vi "ctiSoubor.vi"(8 "PrecistSoubor":bool, 11 "Který soubor chcete otevřít?":path) -> (0 "vystupniError":errorcluster, 2 "Časové razítko souboru:":string, 3 "data":waveform(dbl)[](array[waveform]))   [LabVIEW 2018]
panel:
  # "Vstupy:"
  # "Výstupy:"
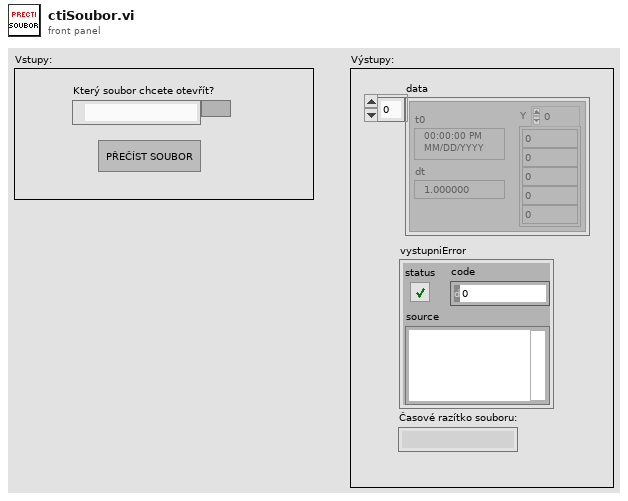
[diagram p1: front panel]
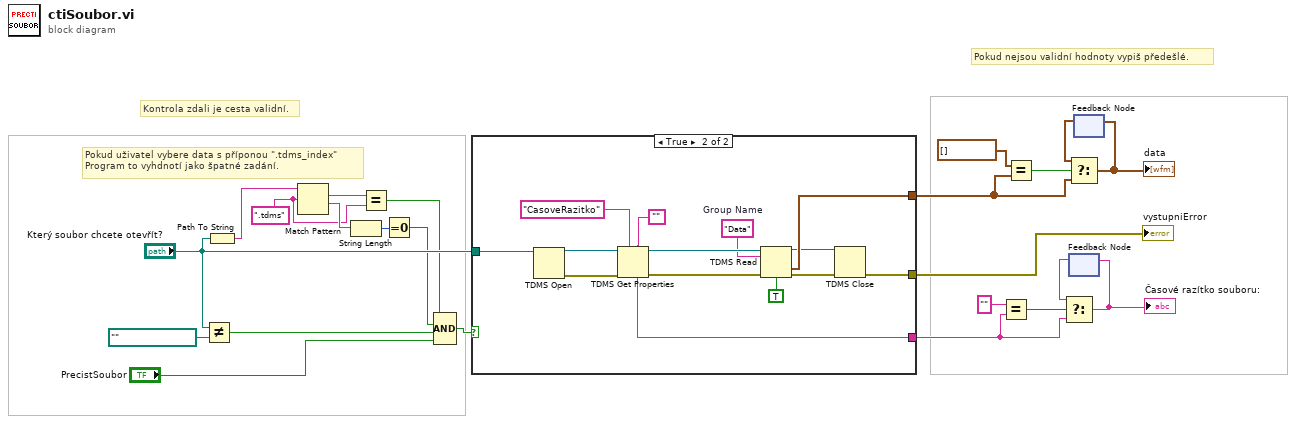
[diagram p0: block diagram]
diagram:
  w2 = ".tdms" ("regular expression")
  # "Pokud uživatel vybere data s příponou \".tdms_index\"\nProgram to vyhdnotí jako špatné zadání."
  # "Kontrola zdali je cesta validní."
  # "Pokud nejsou validní hodnoty vypiš předešlé."
  n1 = Not Equal?(x="Který soubor chcete otevřít?", y=path "" ("Který soubor chcete otevřít?")) -> (x != y?=w7:bool)
  n2 = Path To String(path="Který soubor chcete otevřít?") -> (string=w12:string)
  n3 = Match Pattern(string=w12, regular expression=w2) -> (match substring=w3:string, after substring=w6:string)  [unwired: 1 in, 2 out]
  n4 = String Length(string=w6) -> (length=w5:i32)
  n5 = Equal?(x=w3, y=w2) -> (x = y?=w1:bool)
  n6 = Equal To 0?(x=w5) -> (x = 0?=w4:bool)
  n7 = Compound Arithmetic op=AND(w1, w4, w7, "PrecistSoubor") -> (w10:bool)
  n8 = case shown="True" w10 {
    tunnel: [_ w37] -> w14
    tunnel: [_ w36] -> w20
    tunnel: [_ w35] -> w23
    tunnel: "Který soubor chcete otevřít?" -> [_ w34]
    frame False {
    }
    frame True {
      w28 = "Data"  # Group Name
      n9 = TDMS Open(11:w34) -> (0:w32:errorcluster, 3:w33:refnum<k34>)  [unwired: 6 in]
      n10 = TDMS Get Properties(5:"", 7:"CasoveRazitko" ("element"), 8:w32, 11:w33) -> (0:w30:errorcluster, 3:w31:refnum<k34>, 4:w37:string)  [unwired: 2 in, 3 out]
      n11 = TDMS Read(0:w31, 5:w28, 11:w30, 13:TRUE) -> (4:w24:refnum<k34>, 10:w36:waveform(dbl)[], 15:w25:errorcluster)  [unwired: 4 in, 3 out]
      n12 = TDMS Close(8:w25, 11:w24) -> (0:w35:errorcluster)  [unwired: 1 out]
    }
  }
  "vystupniError" <- w23
  n13 = Equal?(x="", y=w14) -> (x = y?=w17:bool)
  n14 = Equal?(x=waveform(dbl)[] [] ("data"), y=w20) -> (x = y?=w21:bool)
  n15 = feedback #1() -> (w16:string)  [unwired: 1 in]
  n16 = Select(t=w16, s=w17, f=w14) -> (s? t:f=w13:string)
  "Časové razítko souboru:" <- w13
  n17 = feedback-in #1(w13) -> ()
  n18 = feedback #2() -> (w19:waveform(dbl)[])  [unwired: 1 in]
  n19 = Select(t=w19, s=w21, f=w20) -> (s? t:f=w18:waveform(dbl)[])
  "data" <- w18
  n20 = feedback-in #2(w18) -> ()
